vi "Write File Ext.vi"(8 "error in (no error)":errorcluster, 10 "File Ext":string, 11 "File Observer in":refnum<class "File Observer.lvclass">) -> (0 "error out":errorcluster, 3 "File Observer out":refnum<class "File Observer.lvclass">)   [LabVIEW 2015, in "File Observer.lvclass"]
uses:
  File Observer.lvclass
  File Observer.lvclass/File Observer.ctl
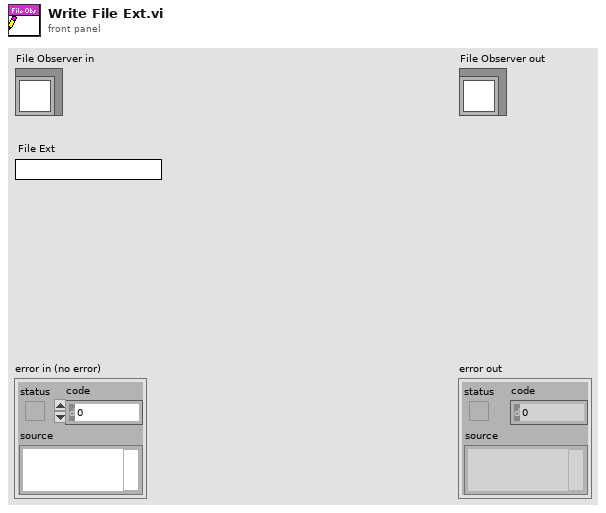
[diagram p1: front panel]
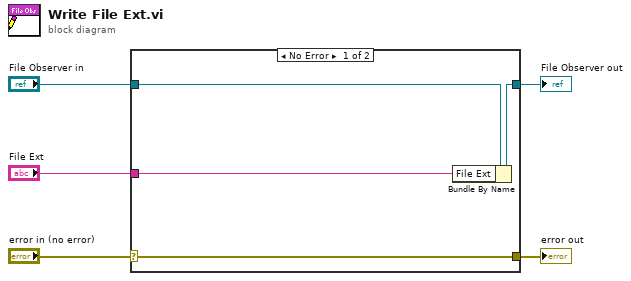
[diagram p0: block diagram]
diagram:
  n1 = case shown="No Error" "error in (no error)" {
    selector: "error in (no error)" -> [w9 w10]
    tunnel: [w9 w10] -> w4
    tunnel: [w7 w11] -> w2
    tunnel: "File Observer in" -> [w8 w11]
    tunnel: "File Ext" -> [w6 _]
    frame No Error {
      n2 = Bundle By Name(cluster=w8, "File Ext"=w6) -> (w7:refnum<class "File Observer.lvclass">)
    }
    frame Error {
    }
  }
  "error out" <- w4
  "File Observer out" <- w2
